vi "Do.vi"(7 "Mediated Asynchronous Actor":refnum<class "Mediated Asynchronous Actor.lvclass">, 8 "error in (no error)":errorcluster, 11 "Parrot Msg in":refnum<class "Parrot Msg.lvclass">) -> (0 "error out":errorcluster, 3 "Parrot Msg out":refnum<class "Parrot Msg.lvclass">, 5 "Mediated Asynchronous Actor out":refnum<class "Mediated Asynchronous Actor.lvclass">)   [LabVIEW 2016, in "Parrot Msg.lvclass"]
doc: "--\nCopyright © 2017 Composed SystemsI All rights reserved.\n\nAuthor: Jon McBee <jon.mcbee@composed.io>\n\nThis library is provided \"AS IS\" ,WITHOUT WARRANTIES OR\nCONDITIONS OF ANY KIND, either express or implied.\n\nComposed Systems -- composed.io\n\nStream 0.0.1.1\nJon McBee - Composed Systems\nCopyright (c) 2017, Composed Systems"
uses:
  <userlib>/Composed Systems/Stream/Sandbox/Async Actor Test/Parrot Msg/Parrot Msg.lvclass
  <userlib>/Composed Systems/Stream/Mediator/Classes/Mediated Asynchronous Actor/Mediated Asynchronous Actor.lvclass
  <userlib>/Composed Systems/Stream/Sandbox/Async Actor Test/Parrot Actor/Parrot.lvclass
  D:/Repos/Stream/software/Mediator/Classes/Mediated Asynchronous Actor/Mediated Asynchronous Actor.lvclass
  <userlib>/Composed Systems/Stream/Sandbox/Async Actor Test/Parrot Msg/Parrot Msg.lvclass/Parrot Msg.ctl
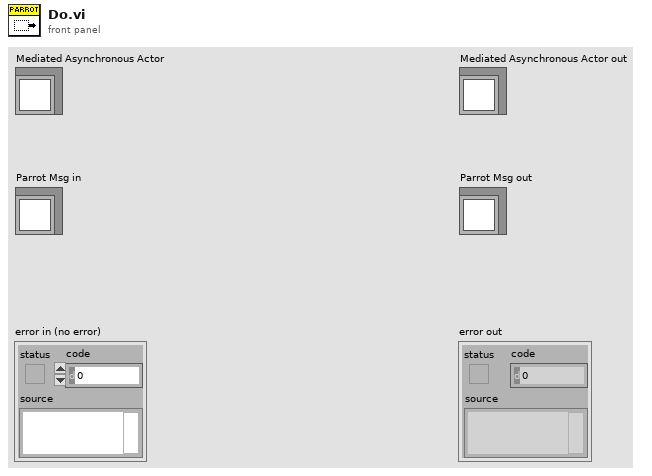
[diagram p1: front panel]
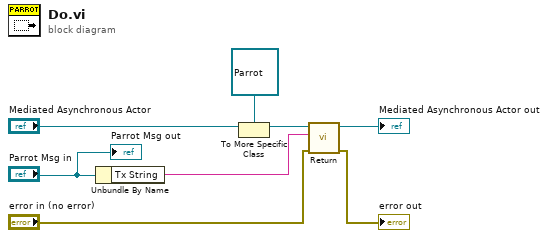
[diagram p0: block diagram]
diagram:
  n1 = Unbundle By Name("Parrot Msg in") -> ("Tx String"=w5:string)
  n2 = To More Specific Class(target class=refnum<class "Parrot.lvclass"> refnum ("Parrot.lvclass"), reference="Mediated Asynchronous Actor") -> (specific class reference=w7:refnum<class "Parrot.lvclass">)  [unwired: 1 in, 1 out]
  n3 = call <userlib>:"Return.vi"("error in (no error)"="error in (no error)", "Tx String"=w5, "Parrot in"=w7) -> ("error out"=→"error out":errorcluster, "Parrot out"=→"Mediated Asynchronous Actor out":refnum<class "Parrot.lvclass">)  [unwired: 7 in]
  "Parrot Msg out" <- "Parrot Msg in"
